vi "LSCI 370 Config Setpoint.vi"(0 "VISA session":refnum<visa-resource-name>, 7 "Setpoint (0.00000E+0)":dbl min=0.0 max=100000000.0 step=1e-06 format="%^.5e", 11 "error in (no error)":errorcluster) -> (4 "dup VISA session":refnum<visa-resource-name>, 15 "error out":errorcluster)   [LabVIEW 2016]
doc: "This VI Configures the setpoint."
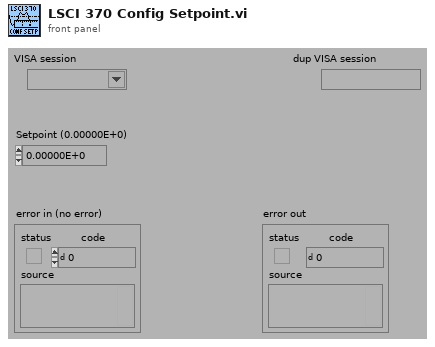
[diagram p1: front panel]
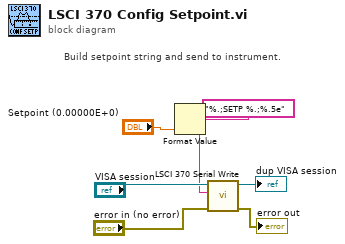
[diagram p0: block diagram]
diagram:
  # "Build setpoint string and send to instrument."
  n1 = Format Value(format string="%.;SETP %.;%.5e", value (0)="Setpoint (0.00000E+0)") -> (output string=w2:string)  [unwired: 1 in]
  n2 = call "LSCI 370 Serial Write.vi"("error in (no error)"="error in (no error)", "Write Buffer (\"\")"=w2, "VISA session"="VISA session") -> ("error out"=→"error out":errorcluster, "dup VISA session"=→"dup VISA session":refnum<visa-resource-name>)  [unwired: 6 in, 1 out]
